vi "OceanOpticsReadOut.vi"() -> ()   [LabVIEW 2015]
uses:
  Maya2000 Typedefs/Maya2000 basic info.ctl
panel:
  out "error out":errorcluster
  out "this maya":T1={"This instruments index"=0, "Name+SerialNumber"="MayaPro2000:MAYP111403", "Number Dark pixels"=8, "NumberOfPixels\nper spectrum"=2068, "NumberOf Maya2000 instrm."=2, "MaximumIntegrationTime\n[us]"=1600000000, "MinimumIntegrationTime\n[us]"=7200}
  in  "number of scans to average":i32=1 min=1 step=1
  out "spectrum":cluster{"Y":dbl[], "Y":dbl[]}[](graph)
  in  "stop":bool
  out "Is saturated?":bool
  in  "integration time [us]":i32=100000
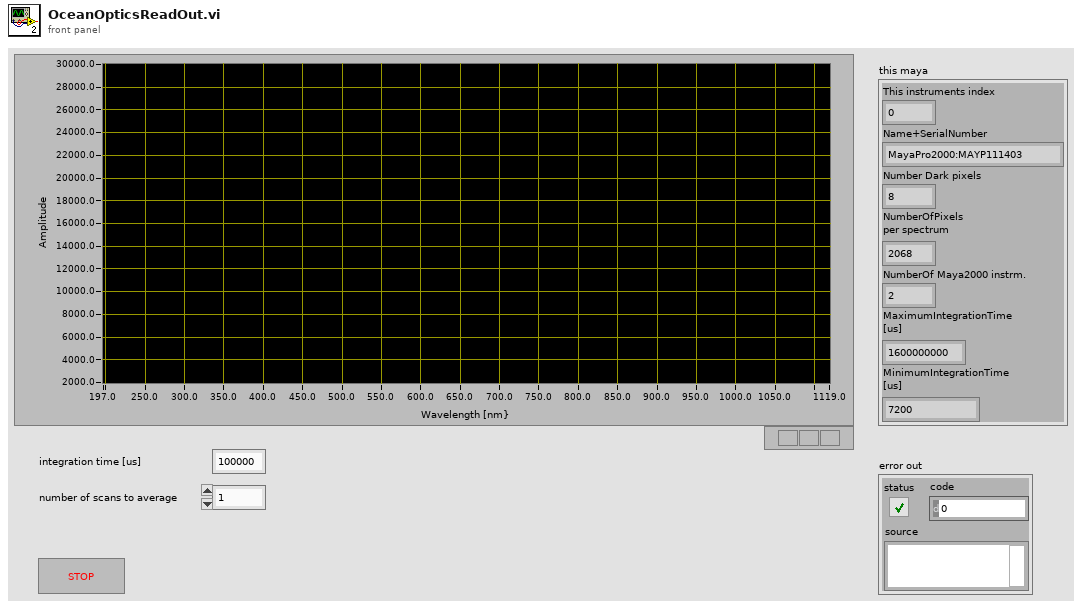
[diagram p1: front panel]
types:
  T1 = typedef "Maya2000 basic info.ctl" = cluster{"This instruments index":i32, "Name+SerialNumber":string, "Number Dark pixels":i32, "NumberOfPixels\nper spectrum":i32, "NumberOf Maya2000 instrm.":i32, "MaximumIntegrationTime\n[us]":i32, "MinimumIntegrationTime\n[us]":i32}
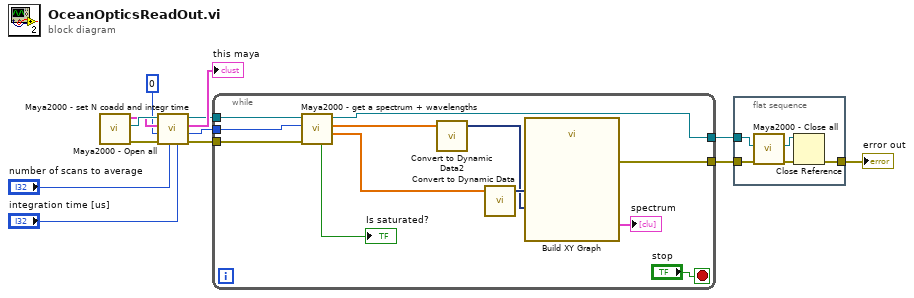
[diagram p0: block diagram]
diagram:
  n1 = call "Maya2000 - Open all.vi"() -> ("error out"=w8:errorcluster, ".NET Refnum out"=w10:refnum<k24>, "Maya2000 Basic \n[UV2400,UV600]"=w9:T1[])  [unwired: 9 in]
  n2 = call "Maya2000 - set N coadd and integr time.vi"("Intgration time\n[us]"="integration time [us]", "numberOfScans\nToAverage"="number of scans to average", "error in (no error)"=w8, "Array index of UV\nspectrometers"=0 ("Intgration time [us] 0"), "Maya2000 basic values"=w9, ".NET Refnum in"=w10) -> ("error out"=w13:errorcluster, "This instruments index"=w3:i32, "This Maya´\nbasic info"=→"this maya":T1, ".NET Refnum out"=w11:refnum<k24>)  [unwired: 2 in]
  n3 = while {
    tunnel: w11 -> [w21]
    tunnel: w13 -> [w20]
    tunnel: w3 -> [w19]
    tunnel: [w22] -> w4
    tunnel: [w14] -> w5
    stop <- "stop" stop-if-true
    n4 = call "Maya2000 - get a spectrum + wavelengths.vi"("error in (no error)"=w20, "This instrments index"=w19, ".NET Refnum in"=w21) -> ("Wavelengths"=w17:dbl[], "Spectrum"=w16:dbl[], ".NET Refnum out"=w14:refnum<k24>, "Is saturated?"=→"Is saturated?":bool)  [unwired: 3 in, 2 out]
    n5 = call "Convert to Dynamic Data2"("Array"=w16) -> ("Dynamic Data Type"=w23:dynamicdata)  [unwired: 3 in]
    n6 = call "Convert to Dynamic Data"("Array"=w17) -> ("Dynamic Data Type"=w24:dynamicdata)  [unwired: 3 in]
    n7 = call "Build XY Graph"("Y Input"=w23, "X Input"=w24) -> ("error out"=w22:errorcluster, "XY Graph"=→"spectrum":cluster{"X":dbl[], "Y":dbl[]}[])  [unwired: 8 in]
  }
  n8 = flat-sequence {
    tunnel: w5 -> [w30]
    tunnel: w4 -> [w29]
    tunnel: [w28] -> w2
    frame #0 {
      n9 = call "Maya2000 - Close all.vi"("error in (no error)"=w29, "Maya reference in"=w30) -> ("error out"=w27:errorcluster, ".NET Refnum out"=w26:refnum<k24>)  [unwired: 8 in]
      n10 = Close Reference(reference=w26, error in (no error)=w27) -> (error out=w28:errorcluster)
    }
  }
  "error out" <- w2
